vi "SLIPsPrint.vi"(0 "listing":string[][](table)) -> ()   [LabVIEW 2010]
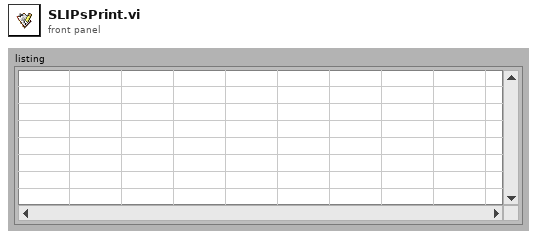
[diagram p1: front panel]
types:
  T1 = typedef "ParamterCluster.ctl" = cluster{"bounce?":bool, "black?":bool, "slide number":i32, "hide?":bool, "selection":bool}
  T2 = typedef "QT_Image.ctl" = cluster{"Width":i32, "Height":i32, "Depth":i32, "data":u8[], "Compressed data":u8[], "Color table":u32[], "Duration":i32, "Options":i32, "Timestamp":i32, "ID":i32, "Reserved":i32, "Dialogs":u32}
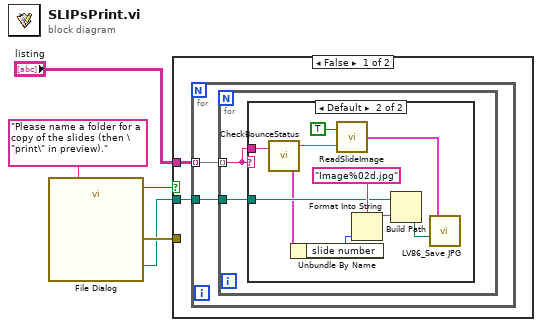
[diagram p0: block diagram]
diagram:
  n1 = call "File Dialog"("prompt"="Please name a folder for a copy of the slides (then \"print\" in preview)." ("element")) -> ("selected path"=w2:path, "cancelled"=w3:bool, "error out"=w5:errorcluster)  [unwired: 11 in, 1 out]
  n2 = case shown="False" w3 {
    tunnel: "listing" -> [w7 _]
    tunnel: w2 -> [w6 _]
    tunnel: w5 -> [_ _]
    frame False {
      n3 = for {
        tunnel: w7 -> [w9] mode=indexing
        tunnel: w6 -> [w8]
        n4 = for {
          tunnel: w9 -> [w11] mode=indexing
          tunnel: w8 -> [w10]
          n5 = case shown="Default" w11 {
            tunnel: w11 -> [_ w21]
            tunnel: w10 -> [_ w17]
            frame "" {
            }
            frame Default {
              n6 = call "CheckBounceStatus.vi"("File Name"=w21) -> ("Parameters"=w15:T1, "file name"=w20:string)  [unwired: 1 in, 1 out]
              n7 = Unbundle By Name(w15) -> ("slide number"=w14:i32)
              n8 = call "ReadSlideImage.vi"("file name"=w20, "Full Size"=TRUE) -> ("Image"=w12:T2)
              n9 = Format Into String(format string="Image%02d.jpg", w14) -> (resulting string=w16:string)  [unwired: 2 in, 1 out]
              n10 = Build Path(base path=w17, name or relative path=w16) -> (appended path=w13:path)
              n11 = call <userlib>:"LV86_Save JPG.vi"("Path to file"=w13, "Image"=w12) -> ()  [unwired: 1 in, 1 out]
            }
          }
        }
      }
    }
    frame True {
    }
  }
